vi "ConnectKRterm.vi"() -> ()   [LabVIEW 2015]
panel:
  out "error out":errorcluster
  in  "stop":bool
  out "standard error":string
  out "return code":i32
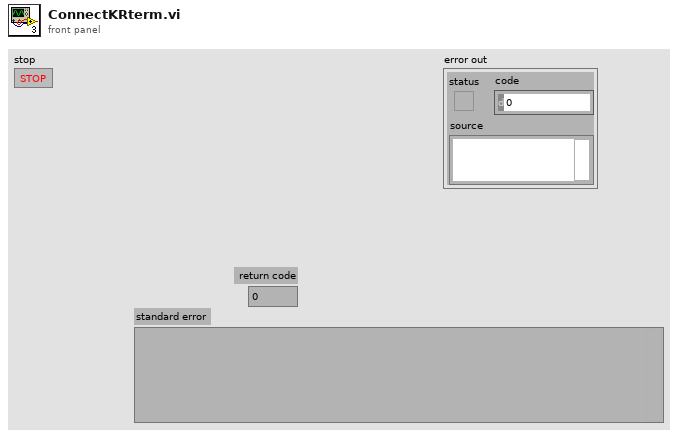
[diagram p1: front panel]
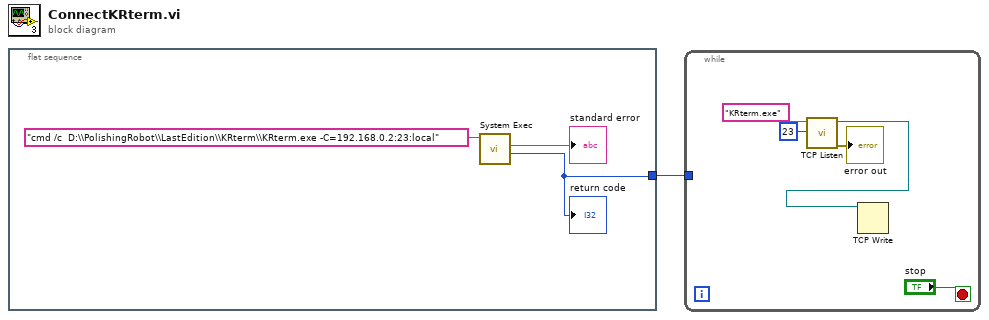
[diagram p0: block diagram]
diagram:
  n1 = flat-sequence {
    tunnel: [w2] -> w1
    frame #0 {
      n2 = call <vilib>:"System Exec.vi"("command line"="cmd /c  D:\\PolishingRobot\\LastEdition\\KRterm\\KRterm.exe -C=192.168.0.2:23:local") -> ("return code"=w2:i32, "standard error"=→"standard error":string)  [unwired: 7 in, 2 out]
      "return code" <- w2
    }
  }
  n3 = while {
    tunnel: w1 -> [_]
    stop <- "stop" stop-if-true
    n4 = call <vilib>:"TCP Listen.vi"("port"=u16 23, "service name"="KRterm.exe") -> ("error out"=→"error out":errorcluster, "connection ID"=w5:refnum<k5>)  [unwired: 5 in, 3 out]
    n5 = TCP Write(connection ID=w5) -> ()  [unwired: 3 in, 3 out]
  }
